vi "Destroy.vi"(0 "reference in":refnum<class "ForecastConditionDisplay.lvclass">, 5 "error in (no error)":errorcluster) -> (14 "reference out":refnum<class "ForecastConditionDisplay.lvclass">, 19 "error out":errorcluster)   [LabVIEW 2020, in "ForecastConditionDisplay.lvclass"]
uses:
  ForecastConditionDisplay.lvclass
  Observer_class/Observer.lvclass
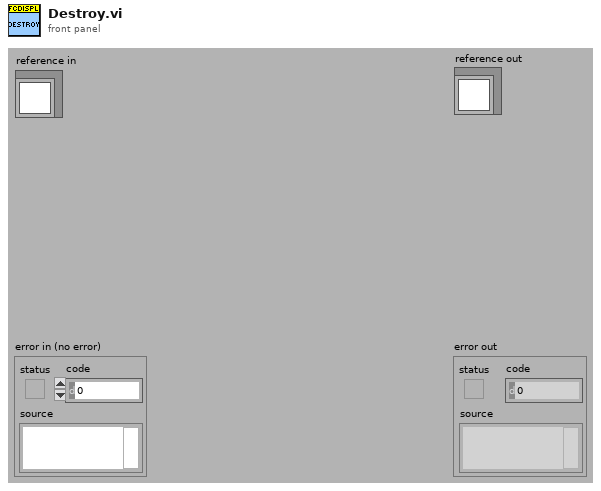
[diagram p1: front panel]
types:
  T1 = typedef "ForecastConditionDisplay.lvclass/ObjectAttributes.ctl" = cluster{"WeatherData":T2}
  T2 = typedef "WeatherData.ctl" = cluster{"Temperature C":dbl, "Humid %":dbl, "Pressure":dbl, "Forecast":string}
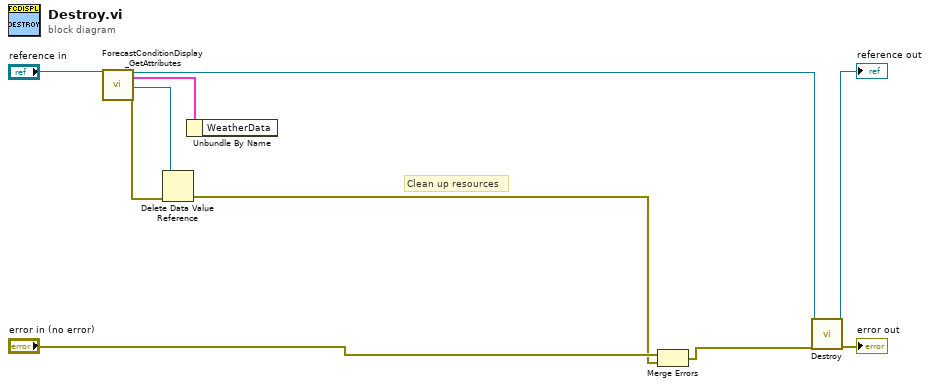
[diagram p0: block diagram]
diagram:
  # "Clean up resources"
  n1 = call "ForecastConditionDisplay_GetAttributes.vi"("reference in"="reference in") -> ("reference out"=w4:refnum<class "ForecastConditionDisplay.lvclass">, "Data"=w7:T1, "DataRef"=w8:refnum<data-value>, "error out"=w9:errorcluster)  [unwired: 15 in]
  n2 = Delete Data Value Reference(data value reference=w8, error in=w9) -> (error out=w5:errorcluster)  [unwired: 1 out]
  n3 = Unbundle By Name(w7) -> ()  [unwired: 1 out]
  n4 = Merge Errors("error in (no error)", w5) -> (w2:errorcluster)
  n5 = call-parent "Destroy.vi"("reference in"=w4, "error in (no error)"=w2) -> ("reference out"=→"reference out":refnum<class "ForecastConditionDisplay.lvclass">, "error out"=→"error out":errorcluster)  [unwired: 16 in]
